vi "RT_read.vi"() -> ()   [LabVIEW 2020]
uses:
  <vilib>/FPGAPlugInAG/cRIO-9054/niLvFpga_Open_cRIO-9054.vi
  <vilib>/Utility/error.llb/Error Cluster From Error Code.vi
  <vilib>/rvi/errors/niLvFpgaAdjustHostInterfaceError.vi
  <vilib>/FPGAPlugInAG/cRIO-9054/niLvFpga_Run_cRIO-9054.vi
  <vilib>/FPGAPlugInAG/cRIO-9054/niLvFpga_Close_cRIO-9054.vi
  <vilib>/rvi/interface/nirviOpenFPGA/nirviOpenFPGA.xnode
  FPGA Bitfiles/basiclogging-fpg_FPGATarget2_FPGA_MzLHMpHrywA.lvbitx
  FPGA.vi
  <vilib>/rvi/interface/nirviMethod/nirviMethod.xnode
  <vilib>/rvi/interface/nirviReadWriteControl/nirviReadWriteControl.xnode
  <vilib>/rvi/interface/nirviCloseFPGA/nirviCloseFPGA.xnode
  <vilib>/rvi/errors/niLvFpgaMergeErrorWithErrorCode.vi
  NiFpgaLv.dll
  <vilib>/FPGAPlugInAG/cRIO-9054/niLvFpga_StartFifo_cRIO-9054.vi
  <vilib>/FPGAPlugInAG/cRIO-9054/niLvFpga_ReadFifo_cRIO-9054.vi
panel:
  out "Actual loop rate (Hz)":dbl
  out "Waveform Graph":sgl[](graph)
  out "Data":fxp<+/-,24,7>[](array[numeric])
  out "Elements Remaining":u32
  in  "Loop number":i32
  out "error out":errorcluster
  out "Timed Out?":bool
  in  "requested Loop rate (Hz)":u32=500
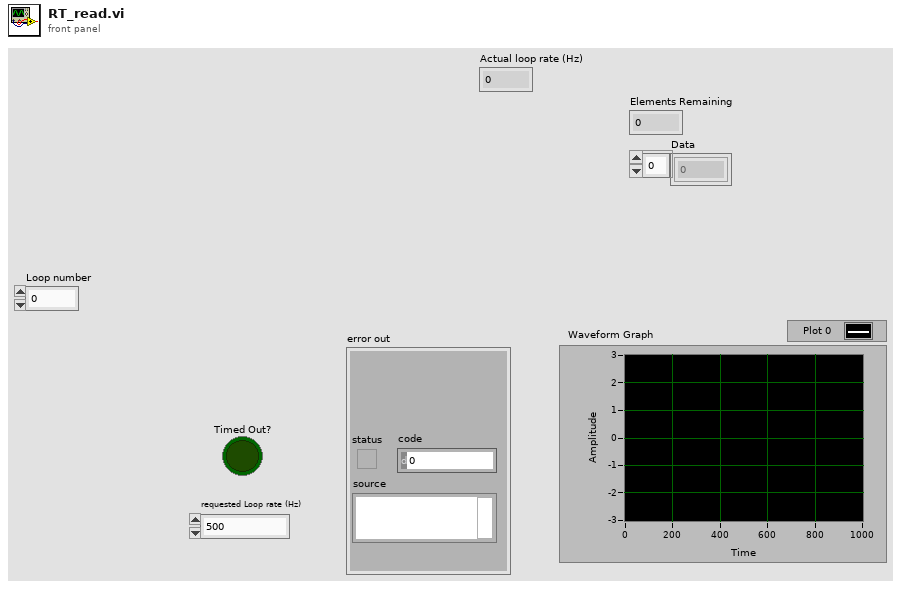
[diagram p1: front panel]
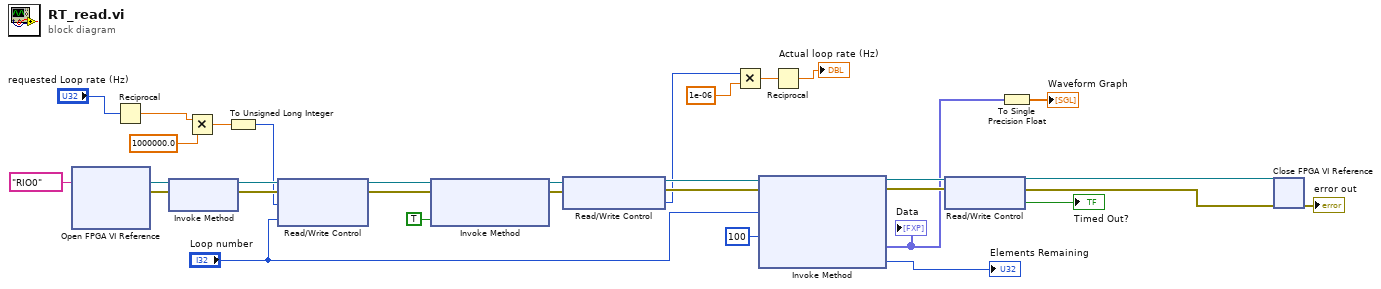
[diagram p0: block diagram]
diagram:
  n1 = xnode "Open FPGA VI Reference"("resource name"=tag "RIO0") -> ("FPGA VI Reference Out"=w29:refnum<k20>, "error out"=w28:errorcluster)  [unwired: 1 in]
  n2 = Reciprocal(x="requested Loop rate (Hz)") -> (1/x=w4:dbl)
  n3 = xnode "Invoke Method"("FPGA VI Reference In"=w29, "error in"=w28) -> ("FPGA VI Reference Out"=w32:refnum<k20>, "error out"=w30:errorcluster)
  n4 = Multiply(x=w4, y=1000000.0) -> (x*y=w2:dbl)
  n5 = To Unsigned Long Integer(number=w2) -> (unsigned 32bit integer=w1:u32)
  n6 = xnode "Read/Write Control"("FPGA VI Reference In"=w32, "error in"=w30, "Rate (uSec)"=w1, "Loop number"="Loop number") -> ("FPGA VI Reference Out"=w31:refnum<k20>, "error out"=w25:errorcluster)
  n7 = xnode "Invoke Method"("FPGA VI Reference In"=w31, "error in"=w25, "Wait Until Done (F)"=TRUE) -> ("FPGA VI Reference Out"=w20:refnum<k20>, "error out"=w19:errorcluster)
  n8 = xnode "Read/Write Control"("FPGA VI Reference In"=w20, "error in"=w19) -> ("FPGA VI Reference Out"=w18:refnum<k20>, "error out"=w17:errorcluster, "Actual loop rate"=w9:u32)
  n9 = Multiply(x=w9, y=1e-06) -> (x*y=w7:dbl)
  n10 = xnode "Invoke Method"("FPGA VI Reference In"=w18, "error in"=w17, "Number of Elements"="Loop number", "Timeout (ms)"=100) -> ("FPGA VI Reference Out"=w16:refnum<k20>, "error out"=w15:errorcluster, "Data"=w11:fxp<+/-,24,7>[], "Elements Remaining"=→"Elements Remaining":u32)
  "Data" <- w11
  n11 = Reciprocal(x=w7) -> (1/x=→"Actual loop rate (Hz)":dbl)
  n12 = xnode "Read/Write Control"("FPGA VI Reference In"=w16, "error in"=w15) -> ("FPGA VI Reference Out"=w27:refnum<k20>, "error out"=w24:errorcluster, "Timed Out?"=→"Timed Out?":bool)
  n13 = To Single Precision Float(number=w11) -> (single precision float=→"Waveform Graph":sgl[])
  n14 = xnode "Close FPGA VI Reference"("FPGA VI Reference In"=w27, "error in"=w24) -> ("error out"=→"error out":errorcluster)
